vi "test - Convert config array - String - 1.vi"(8 "error in (no error)":errorcluster, 11 "TestCase in":refnum<class "Create New Assert Tester.lvclass">) -> (0 "error out":errorcluster, 3 "TestCase out":refnum<class "Create New Assert Tester.lvclass">)   [LabVIEW 2016, in "Create New Assert Tester.lvclass"]
uses:
  Create New Assert Tester.lvclass
  Plugins/Utility/Assert Build Configuration.ctl
  Core/Assert API Components/Failure Actions.ctl
  <vilib>/Utility/Data Type/Type Definitions/Data Type.ctl
  Plugins/Utility/Assert Scripting Configuration.ctl
  <vilib>/addons/_JKI Toolkits/VI Tester/TestCase.llb/TestCase.lvclass
  <vilib>/Utility/Data Type/NI_Data Type.lvlib
  Core/Assert API Components/Assert API Components.lvlib
  C:/Program Files (x86)/National Instruments/LabVIEW 2016/vi.lib/addons/_JKI Toolkits/VI Tester/TestCase.llb/TestCase.lvclass
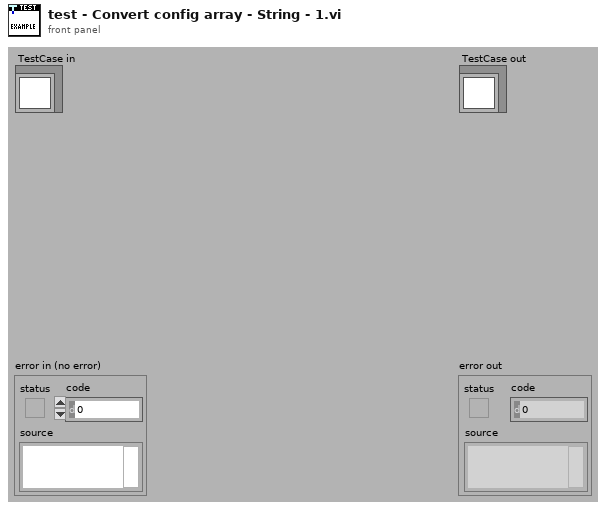
[diagram p1: front panel]
types:
  T1 = typedef "Assert Build Configuration.ctl" = cluster{"Assert Name":string, "Operation":string, "Comparison Value 1":string, "Comparison Value 2":string, "Comment":string, "Default Failure Action":T2, "Description":string, "Operation Display":string, "Active":bool, "Data Type":T3}
  T2 = typedef "Assert API Components.lvlib/Failure Actions.ctl" = enum16{"None", "Log To File", "Pause Execution", "Abort Execution"}
  T3 = typedef "NI_Data Type.lvlib/Data Type.ctl" = enum8{"Invalid Type", "Void", "I8", "I16", "I32", "I64", "U8", "U16", "U32", "U64", "Single Float", "Double Float", "Extended Float", "Single Complex", "Double Complex", "Extended Complex", "Enum U8", "Enum U16", "Enum U32", "Enum U64", "Single Float With Unit", "Double Float With Unit", "Extended Float With Unit", "Single Complex with Unit", "Double Complex with Unit", "Extended Complex with Unit", "Boolean", "String", "Path", "Picture", "Tag", "Array", "Cluster", "Variant", "LV Variant", "Waveform", "Timestamp", "Digital Waveform", "Digital Data", "ExpressData", "Refnum", "External Data", "VI", "Poly VI", "LabVIEW Class Instance", "Fixed Point"}
  T4 = enum16{"None", "Log To File", "Pause Execution", "Abort Execution"}
  T5 = typedef "Assert Scripting Configuration.ctl" = cluster{"Assert Name":string, "Comment":string, "Numeric Operation":string, "Type":T3, "String Operation":string, "DBL Comparison Value 1":dbl, "DBL Comparison Value 2":dbl, "I32 Comparison Value 1":i32, "I32 Comparison Value 2":i32, "Creator":string, "Creation Timestamp":timestamp, "String Comparison Value":string, "Description":string, "Default Failure Action":enum16{"None", "Log To File", "Pause Execution", "Abort Execution"}, "Boolean Comparison Value":bool, "I8 Comparison Value 1":i8, "I8 Comparison Value 2":i8, "I16 Comparison Value 1":i16, "I16 Comparison Value 2":i16, "I64 Comparison Value 1":i64, "I64 Comparison Value 2":i64, "U8 Comparison Value 1":u8, "U8 Comparison Value 2":u8, "U16 Comparison Value 1":u16, "U16 Comparison Value 2":u16, "U32 Comparison Value 1":u32, "U32 Comparison Value 2":u32, "U64 Comparison Value 1":u64, "U64 Comparison Value 2":u64, "EXT Comparison Value 1":ext, "EXT Comparison Value 2":ext, "SGL Comparison Value 1":sgl, "SGL Comparison Value 2":sgl}
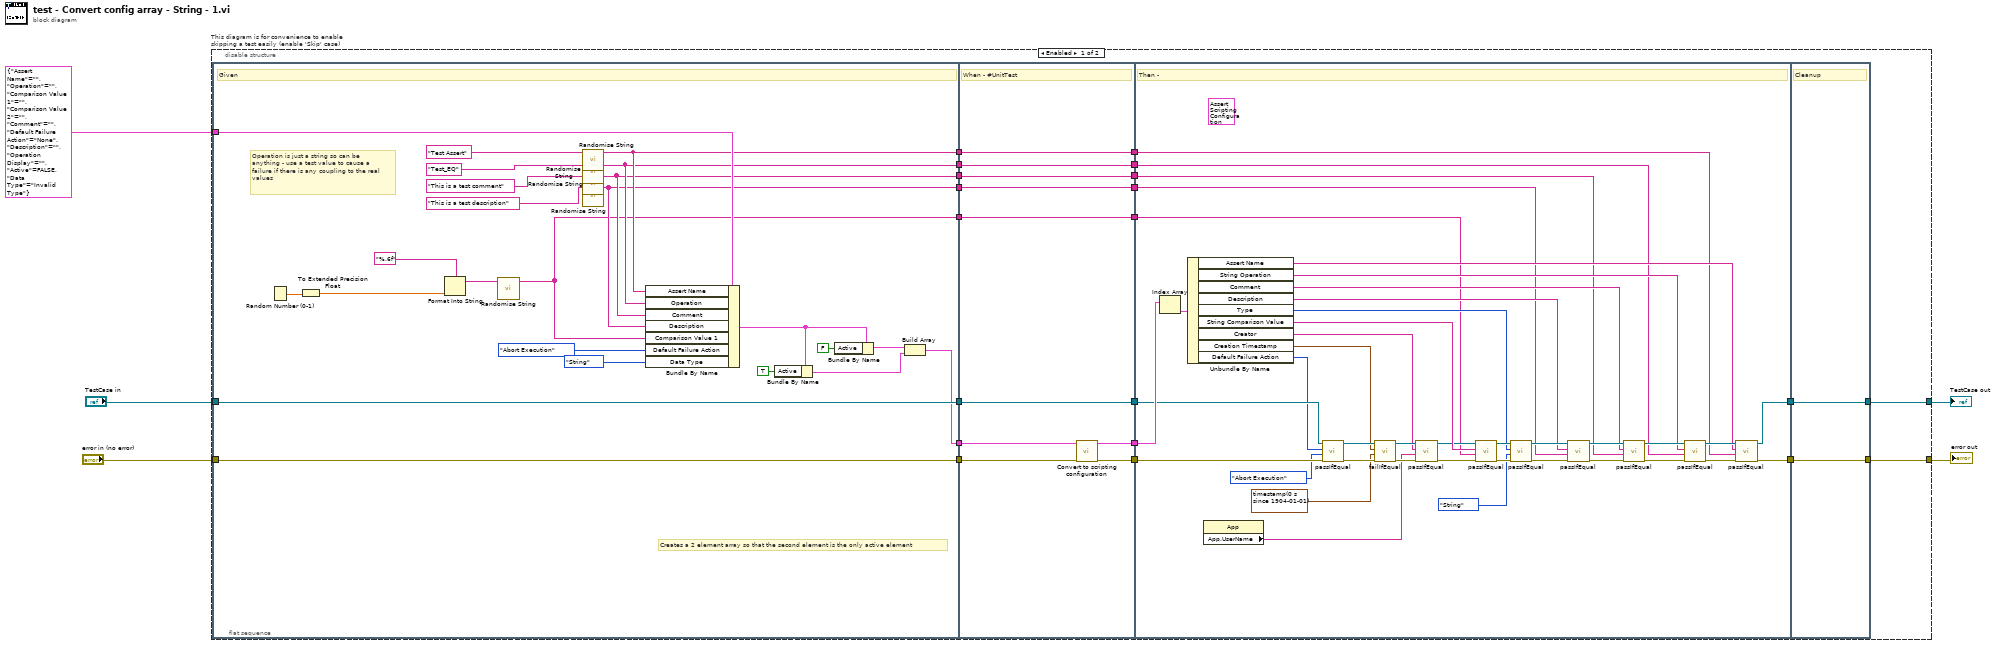
[diagram p0: block diagram]
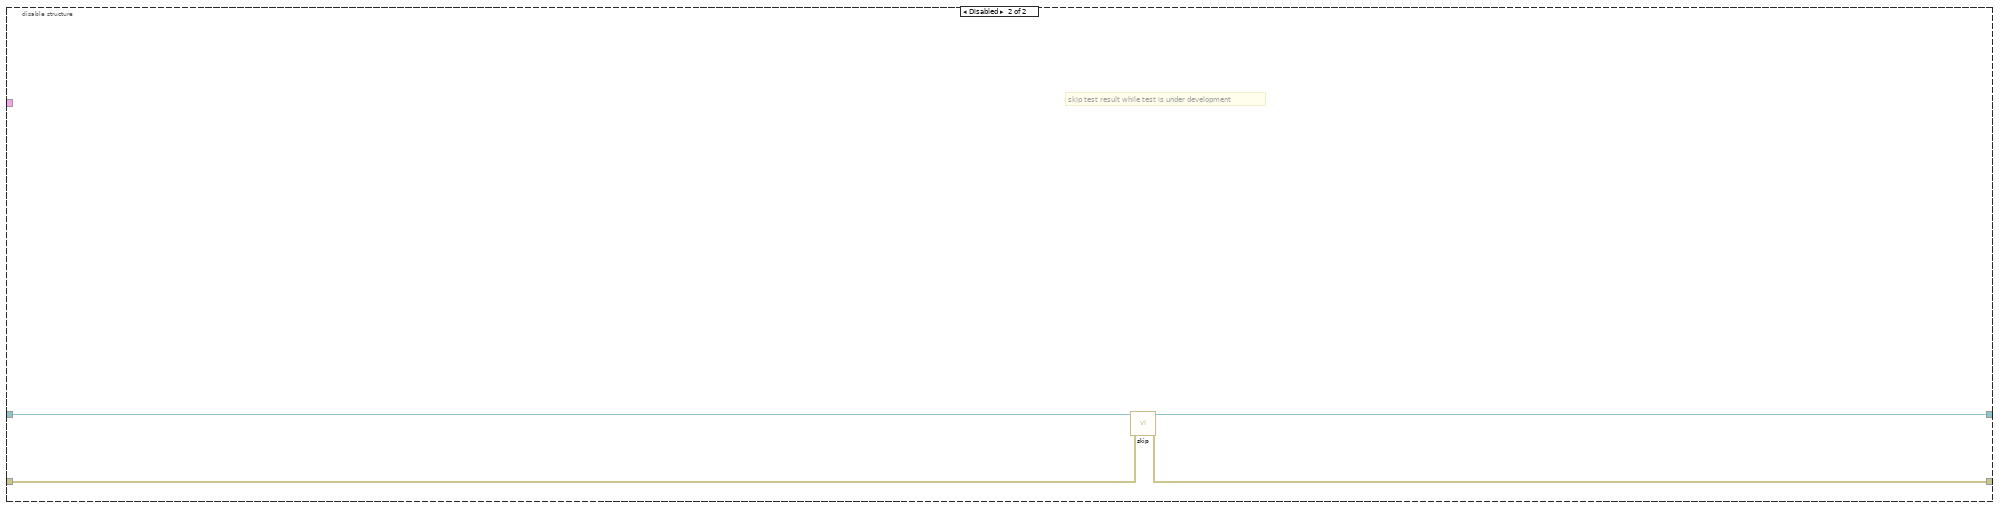
[diagram p2: hidden frame]
diagram:
  n1 = disable-structure "This diagram is for convenience to enable skipping a test easily (enable 'Skip' case)" shown="Enabled" {
    disable-tunnel: "TestCase in" -> [w22 w108]
    disable-tunnel: [w19 w106] -> w2
    disable-tunnel: [w20 w107] -> w4
    disable-tunnel: "error in (no error)" -> [w21 w105]
    disable-tunnel: T1 {"Assert Name"="", "Operation"="", "Comparison Value 1"="", "Comparison Value 2"="", "Comment"="", "Default Failure Action"=enum."None", "Description"="", "Operation Display"="", "Active"=FALSE, "Data Type"=enum."Invalid Type"} ("Assert Build Configuration") -> [w17 _]
    frame Enabled {
      n2 = flat-sequence {
        tunnel: w21 -> [w51]
        tunnel: w22 -> [w52]
        tunnel: [w52] -> w28
        tunnel: [w51] -> w27
        tunnel: w17 -> [w50]
        tunnel: [w45] -> w16
        tunnel: [w37] -> w14
        tunnel: [w36] -> w12
        tunnel: [w35] -> w10
        tunnel: [w34] -> w8
        tunnel: [w29] -> w6
        tunnel: [w62] -> w26
        tunnel: [w60] -> w25
        tunnel: w28 -> [w62]
        tunnel: w27 -> [w61]
        tunnel: [w59] -> w18
        tunnel: w16 -> [w58]
        tunnel: [w57] -> w15
        tunnel: w14 -> [w57]
        tunnel: [w56] -> w13
        tunnel: w12 -> [w56]
        tunnel: [w55] -> w11
        tunnel: w10 -> [w55]
        tunnel: [w54] -> w9
        tunnel: w8 -> [w54]
        tunnel: [w53] -> w7
        tunnel: w6 -> [w53]
        tunnel: [w70] -> w24
        tunnel: [w72] -> w23
        tunnel: w26 -> [w97]
        tunnel: w25 -> [w102]
        tunnel: w18 -> [w100]
        tunnel: w15 -> [w65]
        tunnel: w13 -> [w66]
        tunnel: w11 -> [w67]
        tunnel: w9 -> [w68]
        tunnel: w7 -> [w63]
        tunnel: [w103] -> w20
        tunnel: [w104] -> w19
        tunnel: w24 -> [w104]
        tunnel: w23 -> [w103]
        frame #0 {
          # "Creates a 2 element array so that the second element is the only active element"
          # "Operation is just a string so can be anything - use a test value to cause a failure if there is any coupling to the real values"
          # "Given"
          n3 = Random Number (0-1)() -> (number: 0 to 1=w33:dbl)
          n4 = To Extended Precision Float(1:w33) -> (0:w32:ext)
          n5 = Format Into String(format string="%.6f", w32) -> (resulting string=w31:string)  [unwired: 2 in, 1 out]
          n6 = call "Randomise String.vi"("String in"=w31) -> ("String out"=w29:string)  [unwired: 10 in]
          n7 = call "Randomise String.vi"("String in"="Test Assert" ("Assert Name")) -> ("String out"=w37:string)  [unwired: 10 in]
          n8 = call "Randomise String.vi"("String in"="Test_EQ" ("Operation")) -> ("String out"=w36:string)  [unwired: 10 in]
          n9 = call "Randomise String.vi"("String in"="This is a test comment" ("Comment")) -> ("String out"=w35:string)  [unwired: 10 in]
          n10 = call "Randomise String.vi"("String in"="This is a test description" ("Comment")) -> ("String out"=w34:string)  [unwired: 10 in]
          n11 = Bundle By Name(cluster=w50, "Assert Name"=w37, "Operation"=w36, "Comment"=w35, "Description"=w34, "Comparison Value 1"=w29, "Default Failure Action"=Failure_Actions."Abort Execution", "Data Type"=Data_Type."String") -> (w42:T1)
          n12 = Bundle By Name(cluster=w42, "Active"=TRUE) -> (w40:T1)
          n13 = Bundle By Name(cluster=w42, "Active"=FALSE) -> (w44:T1)
          n14 = Build Array(w44, w40) -> (w45:T1[])
        }
        frame #1 {
          # "When - #UnitTest"
          n15 = call "Convert to scripting configuration.vi"("error in (no error)"=w61, "Multiple Assert Configuration"=w58) -> ("error out"=w60:errorcluster, "Array"=w59:T5[])  [unwired: 7 in, 1 out]
        }
        frame #2 {
          (unwired) T5 {"Assert Name"="", "Comment"="", "Numeric Operation"="", "Type"=enum."Invalid Type", "String Operation"="", "DBL Comparison Value 1"=0.0, "DBL Comparison Value 2"=0.0, "I32 Comparison Value 1"=0, "I32 Comparison Value 2"=0, "Creator"="", "Creation Timestamp"=timestamp(0 s since 1904-01-01), "String Comparison Value"="", "Description"="", "Default Failure Action"=enum."None", "Boolean Comparison Value"=FALSE, "I8 Comparison Value 1"=0, "I8 Comparison Value 2"=0, "I16 Comparison Value 1"=0, "I16 Comparison Value 2"=0, "I64 Comparison Value 1"=0, "I64 Comparison Value 2"=0, "U8 Comparison Value 1"=0, "U8 Comparison Value 2"=0, "U16 Comparison Value 1"=0, "U16 Comparison Value 2"=0, "U32 Comparison Value 1"=0, "U32 Comparison Value 2"=0, "U64 Comparison Value 1"=0, "U64 Comparison Value 2"=0, "EXT Comparison Value 1"=0.0, "EXT Comparison Value 2"=0.0, "SGL Comparison Value 1"=0.0, "SGL Comparison Value 2"=0.0} ("Assert Scripting Configuration")
          # "Then -"
          n16 = Index Array(array=w100) -> (element=w99:T5)  [unwired: 1 in]
          n17 = Unbundle By Name(w99) -> ("Assert Name"=w69:string, "String Operation"=w78:string, "Comment"=w79:string, "Description"=w80:string, "Type"=w81:T3, "String Comparison Value"=w88:string, "Creator"=w89:string, "Creation Timestamp"=w76:timestamp, "Default Failure Action"=w95:T4)
          n18 = property class="App"() -> ("App.UserName"=w74:string)  [unwired: 2 in, 2 out]
          n19 = call-dynamic "passIfEqual.vi"("error in (no error)"=w102, "y"=T4."Abort Execution" ("Default Failure Action"), "x"=w95, "TestCase in"=w97) -> ("error out"=w98:errorcluster, "TestCase out"=w96:refnum<class "Create New Assert Tester.lvclass">)  [unwired: 6 in]
          n20 = call-dynamic "failIfEqual.vi"("error in (no error)"=w98, "y"=timestamp(0 s since 1904-01-01) ("Creation Timestamp"), "x"=w76, "TestCase in"=w96) -> ("error out"=w101:errorcluster, "TestCase out"=w92:refnum<class "Create New Assert Tester.lvclass">)  [unwired: 6 in]
          n21 = call-dynamic "passIfEqual.vi"("error in (no error)"=w101, "y"=w74, "x"=w89, "TestCase in"=w92) -> ("error out"=w93:errorcluster, "TestCase out"=w64:refnum<class "Create New Assert Tester.lvclass">)  [unwired: 6 in]
          n22 = call-dynamic "passIfEqual.vi"("error in (no error)"=w93, "y"=w63, "x"=w88, "TestCase in"=w64) -> ("error out"=w91:errorcluster, "TestCase out"=w86:refnum<class "Create New Assert Tester.lvclass">)  [unwired: 6 in]
          n23 = call-dynamic "passIfEqual.vi"("error in (no error)"=w91, "y"=Data_Type."String" ("Data Type"), "x"=w81, "TestCase in"=w86) -> ("error out"=w87:errorcluster, "TestCase out"=w85:refnum<class "Create New Assert Tester.lvclass">)  [unwired: 6 in]
          n24 = call-dynamic "passIfEqual.vi"("error in (no error)"=w87, "y"=w68, "x"=w80, "TestCase in"=w85) -> ("error out"=w90:errorcluster, "TestCase out"=w83:refnum<class "Create New Assert Tester.lvclass">)  [unwired: 6 in]
          n25 = call-dynamic "passIfEqual.vi"("error in (no error)"=w90, "y"=w67, "x"=w79, "TestCase in"=w83) -> ("error out"=w84:errorcluster, "TestCase out"=w82:refnum<class "Create New Assert Tester.lvclass">)  [unwired: 6 in]
          n26 = call-dynamic "passIfEqual.vi"("error in (no error)"=w84, "y"=w66, "x"=w78, "TestCase in"=w82) -> ("error out"=w94:errorcluster, "TestCase out"=w71:refnum<class "Create New Assert Tester.lvclass">)  [unwired: 6 in]
          n27 = call-dynamic "passIfEqual.vi"("error in (no error)"=w94, "y"=w65, "x"=w69, "TestCase in"=w71) -> ("error out"=w72:errorcluster, "TestCase out"=w70:refnum<class "Create New Assert Tester.lvclass">)  [unwired: 6 in]
        }
        frame #3 {
          # "Cleanup"
        }
      }
    }
    frame Disabled {
      # "skip test result while test is under development"
      n28 = call <vilib>:"skip.vi"("error in (no error)"=w105, "TestCase in"=w108) -> ("error out"=w107:errorcluster, "TestCase out"=w106:refnum<class "Create New Assert Tester.lvclass">)  [unwired: 8 in]
    }
  }
  "error out" <- w4
  "TestCase out" <- w2
